vi "Register AEs.vi"(8 "error in (no error)":errorcluster, 10 "Register Info":T1, 11 "CS++PVMonitor in":refnum<class "CS++PVMonitor.lvclass">) -> (0 "error out":errorcluster, 3 "CS++PVMonitor out":refnum<class "CS++PVMonitor.lvclass">)   [LabVIEW 2015, in "CS++PVMonitor.lvlib" / "CS++PVMonitor.lvclass"]
doc: "Register alarm and event monitoring for process variables."
uses:
  CS++PVMonitor.lvclass
  <vilib>/ActorFramework/Message Enqueuer/Message Enqueuer.lvclass
  CS++PVMonitor Messages/CS++AEUpdate Msg/CS++AEUpdate Msg.lvclass
  CS++PVMonitor Messages/CS++AEUpdate Msg/CS++AEUpdate Msg.lvclass/CS++AEUpdate Msg.ctl
  Classes/CS++ProcessVariables/AlarmEvent/AE.lvclass/AE.ctl
  CS++PVMonitor.lvclass/CS++PVMonitor.ctl
  Classes/CS++ProcessVariables/AlarmEvent/AE.lvclass
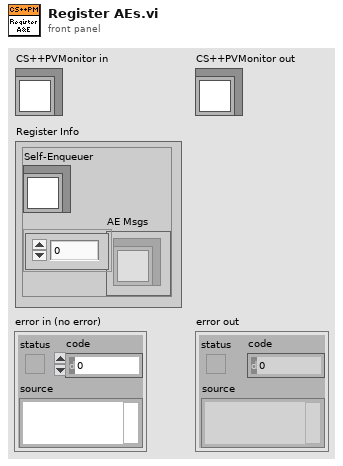
[diagram p1: front panel]
types:
  T1 = cluster{"Self-Enqueuer":refnum<class "Message Enqueuer.lvclass">, "AE Msgs":refnum<class "CS++AEUpdate Msg.lvclass">[]}
  T2 = cluster{"PV URL":string, "Observers":cluster{"Enqueuer":refnum<class "Message Enqueuer.lvclass">, "CS++AEUpdate Msg":refnum<class "CS++AEUpdate Msg.lvclass">}[]}[]
  T3 = cluster{"PV URL":string, "Observers":cluster{"Enqueuer":refnum<class "Message Enqueuer.lvclass">, "CS++AEUpdate Msg":refnum<class "CS++AEUpdate Msg.lvclass">}[]}
  T4 = cluster{"Enqueuer":refnum<class "Message Enqueuer.lvclass">, "CS++AEUpdate Msg":refnum<class "CS++AEUpdate Msg.lvclass">}[]
  T5 = cluster{"Self-Enqueuer":refnum<class "Message Enqueuer.lvclass">, "CS++AEUpdate Msg":refnum<class "CS++AEUpdate Msg.lvclass">}
  T6 = cluster{"Self-Enqueuer":refnum<class "Message Enqueuer.lvclass">, "CS++AEUpdate Msg":refnum<class "CS++AEUpdate Msg.lvclass">}[]
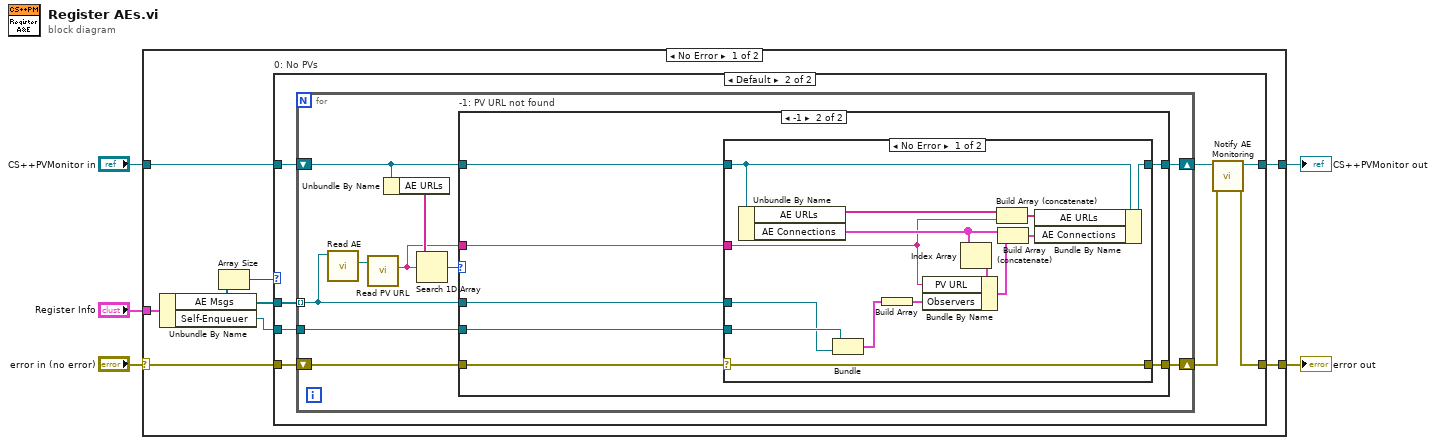
[diagram p0: block diagram]
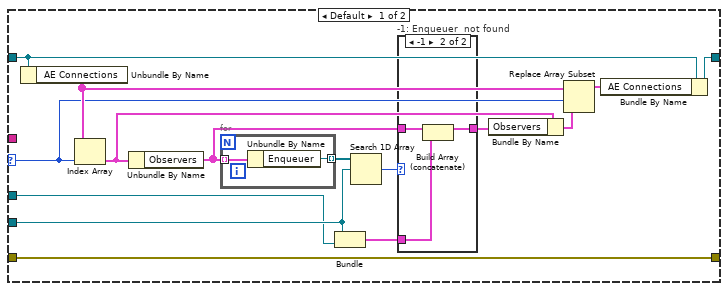
[diagram p3: hidden frame]
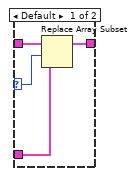
[diagram p4: hidden frame]
diagram:
  n1 = case shown="No Error" "error in (no error)" {
    selector: "error in (no error)" -> [w12 w82]
    tunnel: [w11 w82] -> w4
    tunnel: [w9 w81] -> w2
    tunnel: "CS++PVMonitor in" -> [w10 w81]
    tunnel: "Register Info" -> [w13 _]
    frame No Error {
      n2 = Unbundle By Name(w13) -> ("AE Msgs"=w7:refnum<class "CS++AEUpdate Msg.lvclass">[], "Self-Enqueuer"=w8:refnum<class "Message Enqueuer.lvclass">)
      n3 = Array Size(array=w7) -> (size(s)=w6:i32)
      n4 = case "0: No PVs" shown="Default" w6 {
        tunnel: w7 -> [_ w23]
        tunnel: w12 -> [w14 w22]
        tunnel: [w14 w16] -> w11
        tunnel: w10 -> [w15 w21]
        tunnel: [w15 w18] -> w9
        tunnel: w8 -> [_ w20]
        frame 0 {
        }
        frame Default {
          n5 = for {
            tunnel: w23 -> [w24] mode=indexing
            shift-right: [w28] -> w17
            shift-left: w22 -> [w27]
            shift-right: [w29] -> w19
            shift-left: w21 -> [w31]
            tunnel: w20 -> [w30]
            n6 = call "Read AE.vi"("CS++AEUpdate Msg in"=w24) -> ("AE"=w26:refnum<class "AE.lvclass">)  [unwired: 8 in, 2 out]
            n7 = call "Read PV URL.vi"("AE in"=w26) -> ("PV URL"=w25:string)  [unwired: 8 in, 2 out]
            n8 = Unbundle By Name(w31) -> ("AE URLs"=w33:string[])
            n9 = Search 1D Array(1D array=w33, element=w25) -> (index of element=w32:i32)  [unwired: 1 in]
            n10 = case "-1: PV URL not found" shown="-1" w32 {
              selector: w32 -> [w43 _]
              tunnel: w31 -> [w47 w59]
              tunnel: w30 -> [w40 w63]
              tunnel: w24 -> [w34 w62]
              tunnel: [w45 w64] -> w29
              tunnel: [w42 w61] -> w28
              tunnel: w27 -> [w42 w58]
              tunnel: w25 -> [_ w60]
              frame Default {
                n11 = Unbundle By Name(w47) -> ("AE Connections"=w44:T2)
                n12 = Index Array(array=w44, index=w43) -> (element=w41:T3)
                n13 = Unbundle By Name(w41) -> ("Observers"=w46:T4)
                n14 = for {
                  tunnel: w46 -> [w57] mode=indexing
                  tunnel: [w56] -> w48 mode=indexing
                  n15 = Unbundle By Name(w57) -> ("Enqueuer"=w56:refnum<class "Message Enqueuer.lvclass">)
                }
                n16 = Bundle("Self-Enqueuer"=w40, "CS++AEUpdate Msg"=w34) -> (w39:T5)  [unwired: 1 in]
                n17 = Search 1D Array(1D array=w48, element=w40) -> (index of element=w35:i32)  [unwired: 1 in]
                n18 = case "-1: Enqueuer  not found" shown="-1" w35 {
                  selector: w35 -> [w49 _]
                  tunnel: w46 -> [w52 w55]
                  tunnel: w39 -> [w51 w53]
                  tunnel: [w50 w54] -> w37
                  frame Default {
                    n19 = Replace Array Subset(array=w52, new element=w51, index=w49) -> (w50:T4)
                  }
                  frame -1 {
                    n20 = Build Array (concatenate)(w55, w53) -> (w54:T6)
                  }
                }
                n21 = Bundle By Name(cluster=w41, "Observers"=w37) -> (w36:T3)
                n22 = Replace Array Subset(array=w44, new element=w36, index=w43) -> (w38:T2)
                n23 = Bundle By Name(cluster=w47, "AE Connections"=w38) -> (w45:refnum<class "CS++PVMonitor.lvclass">)
              }
              frame -1 {
                n24 = case shown="No Error" w58 {
                  selector: w58 -> [w66 w79]
                  tunnel: [w78 w80] -> w64
                  tunnel: w63 -> [w75 _]
                  tunnel: w62 -> [w65 _]
                  tunnel: w59 -> [w70 w80]
                  tunnel: w60 -> [w68 _]
                  tunnel: [w66 w79] -> w61
                  frame No Error {
                    n25 = Unbundle By Name(w70) -> ("AE URLs"=w67:string[], "AE Connections"=w77:T2)
                    n26 = Bundle("Self-Enqueuer"=w75, "CS++AEUpdate Msg"=w65) -> (w74:T5)  [unwired: 1 in]
                    n27 = Build Array(w74) -> (w72:T6)
                    n28 = Index Array(array=w77) -> (element=w76:T3)  [unwired: 1 in]
                    n29 = Bundle By Name(cluster=w76, "PV URL"=w68, "Observers"=w72) -> (w71:T3)
                    n30 = Build Array (concatenate)(w67, w68) -> (w69:string[])
                    n31 = Build Array (concatenate)(w77, w71) -> (w73:T2)
                    n32 = Bundle By Name(cluster=w70, "AE URLs"=w69, "AE Connections"=w73) -> (w78:refnum<class "CS++PVMonitor.lvclass">)
                  }
                  frame Error {
                  }
                }
              }
            }
          }
          n33 = call-dynamic "Notify AE Monitoring.vi"("error in (no error)"=w17, "CS++PVMonitor in"=w19) -> ("error out"=w16:errorcluster, "CS++PVMonitor out"=w18:refnum<class "CS++PVMonitor.lvclass">)  [unwired: 8 in]
        }
      }
    }
    frame Error {
    }
  }
  "error out" <- w4
  "CS++PVMonitor out" <- w2
